vi "Test Kinect.vi"() -> ()   [LabVIEW 2015]
uses:
  Controls/Led Control.ctl
  Controls/Video Resolution Control.ctl
  Controls/Video Format Control.ctl
  <vilib>/Analysis/baseanly.llb/Mean (DBL).vi
  <vilib>/myRIO/Common/Instrument Driver Framework/myRIO v1.0/UART/vis/myRIO v1.0 Close UART.vi
  <vilib>/myRIO/Common/Instrument Driver Framework/Utilities/vis/FPGA Ref Manager.vi
  <vilib>/myRIO/Common/Instrument Driver Framework/myRIO v1.0/myRIO v1.0 Reset FPGA.vi
  <vilib>/myRIO/Common/Instrument Driver Framework/myRIO v1.0/IRQ/vis/myRIO v1.0 IRQ Info FGV.vi
  <vilib>/myRIO/Common/Instrument Driver Framework/myRIO v1.0/IRQ/vis/myRIO v1.0 Timer IRQ Info FGV.vi
  <vilib>/myRIO/Common/Instrument Driver Framework/myRIO v1.0/IRQ/vis/myRIO v1.0 ISR Agent.vi
  <vilib>/myRIO/Instrument Drivers/Utilities/Utilities.lvlib
  <vilib>/Analysis/NI_AALBase.lvlib
panel:
  out "Video":T1(plugin-control)
  in  "Video Res":T2=enum."FREENECT_RESOLUTION_MEDIUM"
  out "error out":errorcluster
  out "mean":dbl format="%0.2f"
  in  "Size":enum16{"Low (320x240)", "Tiny (160x120)"}(ring)
  out "Depth":T1(plugin-control)
  in  "stop":bool
  out "period":u32
  in  "Depth Format":T3(ring)
  in  "tilt degree":i32=12
  in  "Led Option":T4=enum."LED_RED"
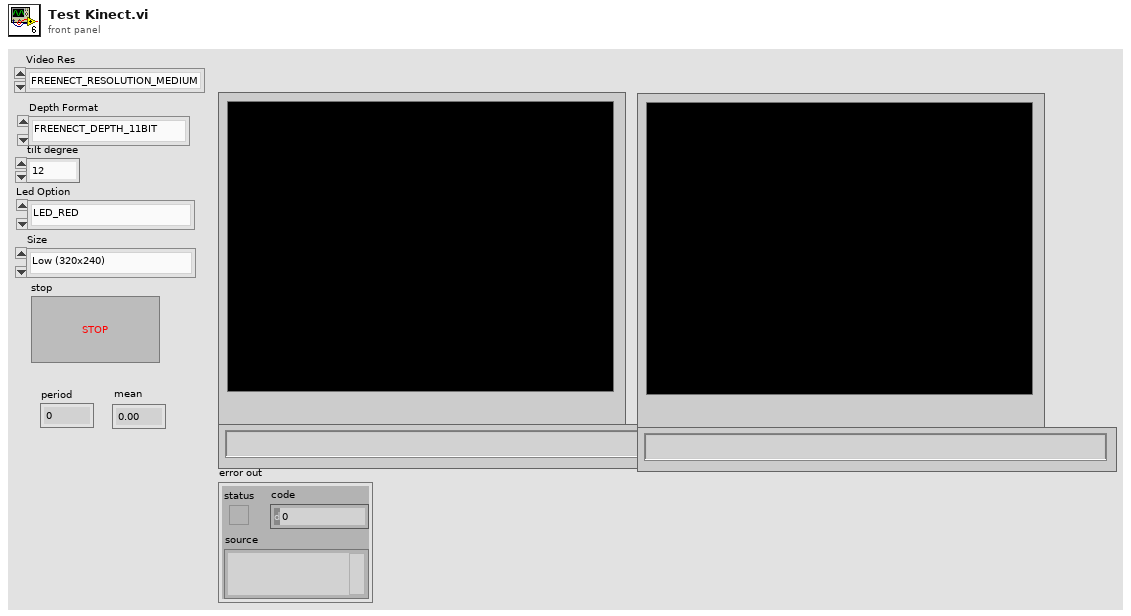
[diagram p1: front panel]
types:
  T1 = typedef "IMAQ Image.ctl" = refnum<image>
  T2 = typedef "Video Resolution Control.ctl" = enum32{"FREENECT_RESOLUTION_LOW", "FREENECT_RESOLUTION_MEDIUM", "FREENECT_RESOLUTION_HIGH"}
  T3 = enum32{"FREENECT_DEPTH_11BIT", "FREENECT_DEPTH_10BIT", "FREENECT_DEPTH_11BIT_PACKED", "FREENECT_DEPTH_10BIT_PACKED", "FREENECT_DEPTH_REGISTERED", "FREENECT_DEPTH_MM"}
  T4 = typedef "Led Control.ctl" = enum32{"LED_OFF", "LED_GREEN", "LED_RED", "LED_YELLOW", "LED_BLINK_GREEN", "LED_BLINK_GREEN2", "LED_BLINK_RED_YELLOW"}
  T5 = typedef "Video Format Control.ctl" = enum32{"FREENECT_VIDEO_RGB", "FREENECT_VIDEO_BAYER", "FREENECT_VIDEO_IR_8BIT", "FREENECT_VIDEO_IR_10BIT", "FREENECT_VIDEO_IR_10BIT_PACKED", "FREENECT_VIDEO_YUV_RGB", "FREENECT_VIDEO_YUV_RAW"}
  T6 = typedef "Image Type" = u32
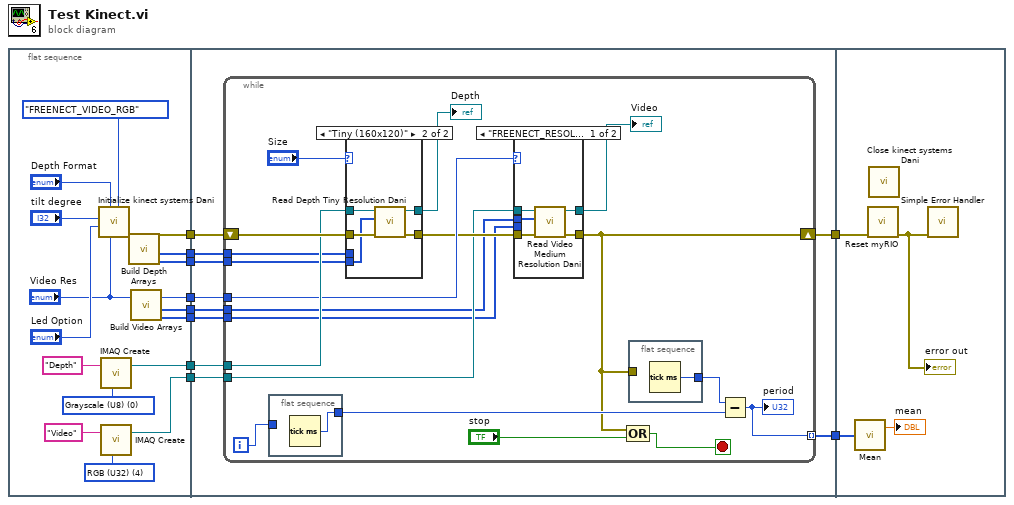
[diagram p0: block diagram]
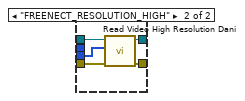
[diagram p2: hidden frame]
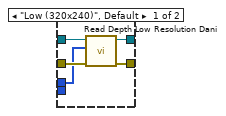
[diagram p3: hidden frame]
diagram:
  n1 = flat-sequence {
    tunnel: [w26] -> w10
    tunnel: [w25] -> w9
    tunnel: [w19] -> w8
    tunnel: [w18] -> w7
    tunnel: [w16] -> w4
    tunnel: [w15] -> w3
    tunnel: ["Video Res"] -> w2
    tunnel: [w11] -> w1
    tunnel: w10 -> [w36]
    tunnel: [w35] -> w6
    tunnel: w9 -> [w34]
    tunnel: w8 -> [w33]
    tunnel: w7 -> [w32]
    tunnel: [w31] -> w5
    tunnel: w4 -> [w28]
    tunnel: w3 -> [w27]
    tunnel: w2 -> [w30]
    tunnel: w1 -> [w29]
    tunnel: w6 -> [w81]
    tunnel: w5 -> [w79]
    frame #0 {
      w13 = T6 4 items=["Grayscale (U8)", "Grayscale (I16)", "Grayscale (SGL)", "Complex (CSG)", "RGB (U32)", "HSL (U32)", "RGB (U64)", "Grayscale (U16)"] ("Image Type")
      w20 = T6 0 items=["Grayscale (U8)", "Grayscale (I16)", "Grayscale (SGL)", "Complex (CSG)", "RGB (U32)", "HSL (U32)", "RGB (U64)", "Grayscale (U16)"] ("Image Type")
      n2 = call "Initialize kinect systems Dani.vi"("Video Format"=Video_Format_Control."FREENECT_VIDEO_RGB", "Video Res"="Video Res", "Depth Format"="Depth Format", "Led Option"="Led Option", "tilt degree"="tilt degree") -> ("error out"=w26:errorcluster)  [unwired: 6 in]
      n3 = call "IMAQ Create"("Image Name"="Depth", "Image Type"=w20) -> ("New Image"=w25:T1)  [unwired: 3 in, 1 out]
      n4 = call "IMAQ Create"("Image Name"="Video", "Image Type"=w13) -> ("New Image"=w11:T1)  [unwired: 3 in, 1 out]
      n5 = call "Build Depth Arrays.vi"() -> ("Array Tiny"=w18:u16[], "Array Low"=w19:u16[])  [unwired: 10 in]
      n6 = call "Build Video Arrays.vi"() -> ("Array High"=w15:u32[], "Array Medium"=w16:u32[])  [unwired: 9 in, 1 out]
    }
    frame #1 {
      n7 = while {
        shift-right: [w37] -> w35
        shift-left: w36 -> [w53]
        tunnel: w34 -> [w50]
        tunnel: w33 -> [w49]
        tunnel: w32 -> [w48]
        tunnel: [w44] -> w31 mode=indexing
        tunnel: w30 -> [w43]
        tunnel: w29 -> [w41]
        tunnel: w28 -> [w40]
        tunnel: w27 -> [w39]
        i -> [w47]
        stop <- w51 stop-if-true
        n8 = flat-sequence {
          tunnel: w47 -> [_]
          tunnel: [w67] -> w45
          frame #0 {
            n9 = Tick Count (ms)() -> (millisecond timer value=w67:u32)
          }
        }
        n10 = case shown="\"Tiny (160x120)\"" "Size" {
          tunnel: [w72 w77] -> w54
          tunnel: [w71 w75] -> w42
          tunnel: w53 -> [w70 w76]
          tunnel: w50 -> [w69 w74]
          tunnel: w49 -> [w68 _]
          tunnel: w48 -> [_ w73]
          frame "Low (320x240)", Default {
            n11 = call "Read Depth Low Resolution Dani.vi"("error in (no error)"=w70, "depth"=w68, "Image In"=w69) -> ("error out"=w71:errorcluster, "Image Out"=w72:T1)  [unwired: 7 in]
          }
          frame "Tiny (160x120)" {
            n12 = call "Read Depth Tiny Resolution Dani.vi"("error in (no error)"=w76, "depth"=w73, "Image In"=w74) -> ("error out"=w75:errorcluster, "Image Out"=w77:T1)  [unwired: 7 in]
          }
        }
        "Depth" <- w54
        n13 = case shown="\"FREENECT_RESOLUTION_MEDIUM\", Default" w43 {
          tunnel: w42 -> [w60 w63]
          tunnel: w41 -> [w59 w65]
          tunnel: w40 -> [w58 _]
          tunnel: w39 -> [_ w64]
          tunnel: [w56 w62] -> w37
          tunnel: [w57 w61] -> w38
          frame "FREENECT_RESOLUTION_MEDIUM", Default {
            n14 = call "Read Video Medium Resolution Dani.vi"("error in (no error)"=w60, "video"=w58, "Image In"=w59) -> ("error out"=w56:errorcluster, "Image Out"=w57:T1)  [unwired: 7 in]
          }
          frame "FREENECT_RESOLUTION_HIGH" {
            n15 = call "Read Video High Resolution Dani.vi"("error in (no error)"=w63, "video"=w64, "Image In"=w65) -> ("error out"=w62:errorcluster, "Image Out"=w61:T1)  [unwired: 7 in]
          }
        }
        "Video" <- w38
        n16 = Compound Arithmetic op=OR(w37, "stop") -> (w51:bool)
        n17 = flat-sequence {
          tunnel: [w66] -> w46
          tunnel: w37 -> [_]
          frame #0 {
            n18 = Tick Count (ms)() -> (millisecond timer value=w66:u32)
          }
        }
        n19 = Subtract(x=w46, y=w45) -> (x-y=w44:u32)
        "period" <- w44
      }
    }
    frame #2 {
      n20 = call-poly <vilib>:"Mean.vi"("X"=w79) -> ("mean"=→"mean":dbl)  [unwired: 1 out]
      n21 = call <vilib>:"Reset myRIO.vi"("error in (no error)"=w81) -> ("error out"=w80:errorcluster)  [unwired: 10 in]
      "error out" <- w80
      n22 = call "Close kinect systems Dani.vi"() -> ()  [unwired: 11 in, 1 out]
      n23 = call <vilib>:"Simple Error Handler.vi"("error in (no error)"=w80) -> ()  [unwired: 4 in, 5 out]
    }
  }
